vi "CR-导丝纤维毛发检测2.vi"(8 "error in (no error)":errorcluster caption="错误输入（无错误）", 11 "名称或相对路径":string="Template Program") -> (0 "error in (no error) 2":errorcluster caption="错误输入（无错误）")   [LabVIEW 2017]
uses:
  Global System.vi
  <vilib>/Utility/xml.llb/Write to XML File(string).vi
  Picture/SaveButtom.ctl
  <vilib>/vision/Pattern Matching.llb/IMAQ Curve Parameters.ctl
  <vilib>/userdefined/High Color/IMAQdx.ctl
panel:
  in  "相机选择":T1="cam0" caption="Session Out CCD3"
  in  "获取图像":bool
  in  "ROI获取":bool
  in  "创建模板":bool
  in  "保存图像":bool
  out "添加的路径":path
  in  "刷新":bool
  in  "测试按钮":bool
  in  "保存按钮":bool
  in  "Main":enum32{"主参数", "模板匹配参数 ", "测试效果"}(tab)
  in  "导丝纤维毛发检测2基础参数":T2={"IsNorImage"=TRUE, "Exposure Values"=100289, "ImagePath"=path "C:/Users/hedongpo/Desktop/514-hdp/Alignment Assemble System/Test Picture/B/3.bmp"} caption="参数界面" {"Exposure Values" scale=0.0..200000.0}
  in  "导丝纤维毛发检测2参数":T4={"Max Number"=11.0, "Curve Extraction Settings "={"Extraction Mode"=0, "Edge Threshold"=25, "Edge Filter Size"=1, "Min Length"=19, "Row Search Step Size"=5, "Col Search Step Size"=5, "Max Endpoint Gap"=10, "Closed"=FALSE, "Subpixel"=FALSE}, "Color Mode (Histogram 1)"=0, "Range (Threshold 1)"={"Lower value"=62.0, "Upper value"=255.0}, "Clamp Settings (Max Clamp 1)"={"Angle Range (+/-)"=10.0, "Edge Polarity"={"Start"=0, "End"=0}}} {"Clamp Settings (Max Clamp 1)"."Edge Polarity"."Start" items=["Any", "Rising", "Falling"]; "Clamp Settings (Max Clamp 1)"."Edge Polarity"."End" items=["Any", "Rising", "Falling"]; "Color Mode (Histogram 1)" items=["RGB", "HSL", "HSV", "HSI"]; "Curve Extraction Settings"."Extraction Mode" items=["Normal", "Uniform Regions"]; "Curve Extraction Settings"."Edge Filter Size" items=["Fine", "Normal", "Contour Tracing"]; "Curve Extraction Settings"."Max Endpoint Gap" min=0; "Curve Extraction Settings"."Col Search Step Size" min=1 max=255 step=1; "Curve Extraction Settings"."Row Search Step Size" min=1 max=255 step=1; "Curve Extraction Settings"."Min Length" min=0; "Curve Extraction Settings"."Edge Threshold" min=1 max=350 step=1}
  out "结果":bool
  out "原始图像":T5(plugin-control)
  out "路径输出":path
  in  "Vision Paramter Save Buttom":T6
  out "system time":string
  in  "取消按钮":bool
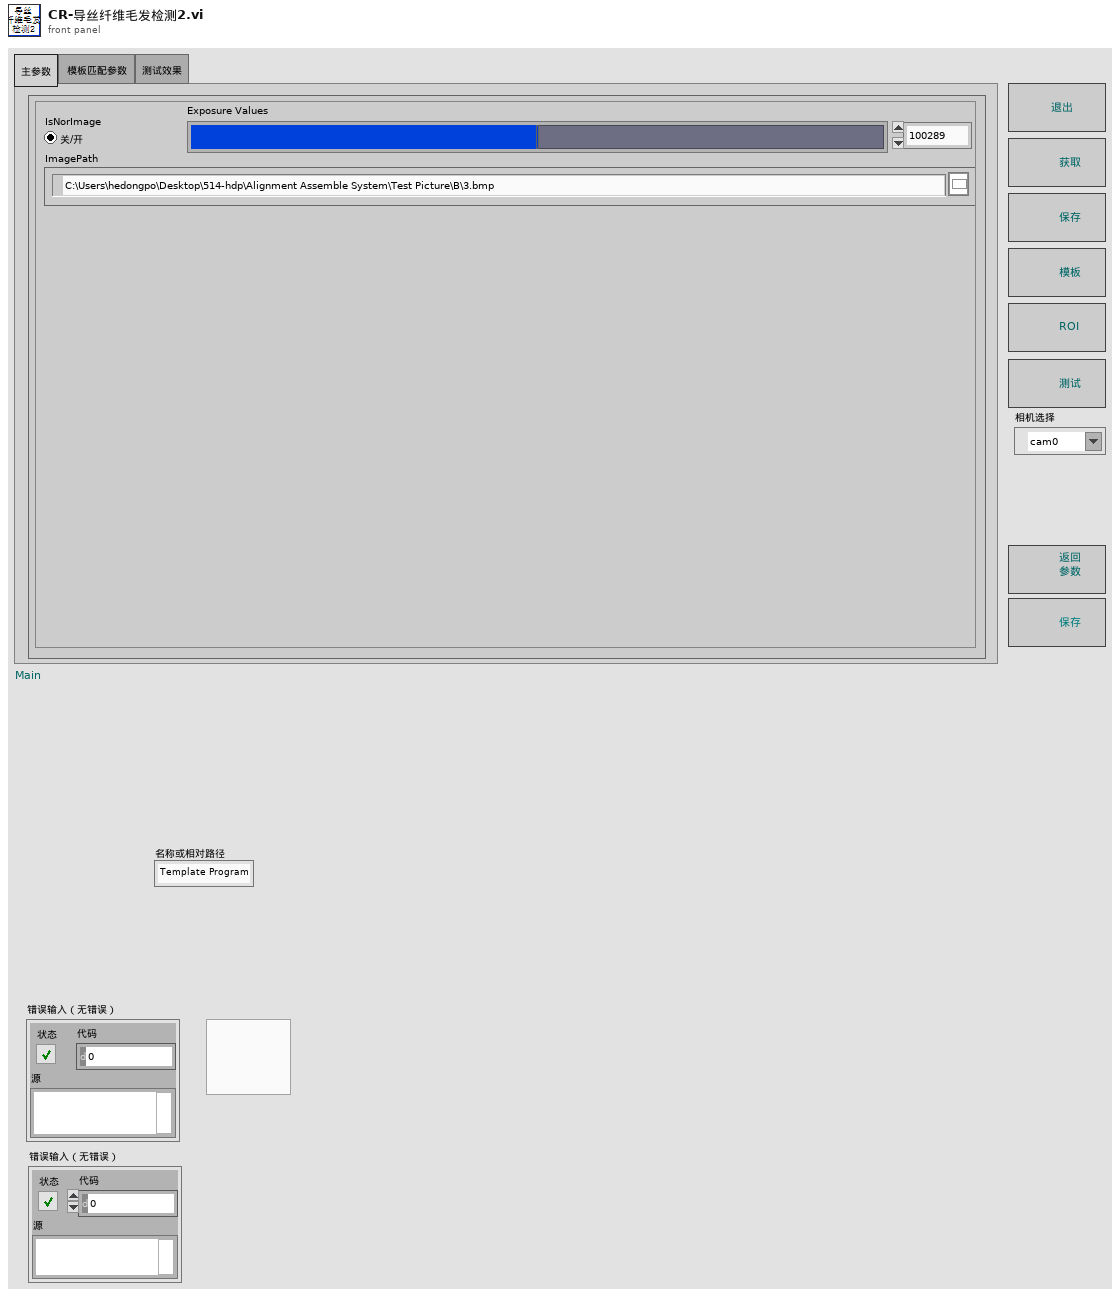
[diagram p1: front panel]
types:
  T1 = typedef "IMAQdx.ctl" = refnum<k21>
  T2 = cluster{"IsNorImage":bool, "Exposure Values":u32, "ImagePath":path}
  T3 = typedef "IMAQ Curve Parameters.ctl" = cluster{"Extraction Mode":u32, "Edge Threshold":i32, "Edge Filter Size":u32, "Min Length":i32, "Row Search Step Size":i32, "Col Search Step Size":i32, "Max Endpoint Gap":i32, "Closed":bool, "Subpixel":bool}
  T4 = cluster{"Max Number":sgl, "Curve Extraction Settings ":T3, "Color Mode (Histogram 1)":u16, "Range (Threshold 1)":cluster{"Lower value":sgl, "Upper value":sgl}, "Clamp Settings (Max Clamp 1)":cluster{"Angle Range (+/-)":dbl, "Edge Polarity":cluster{"Start":u32, "End":u32}}}
  T5 = typedef "IMAQ Image.ctl" = refnum<image>
  T6 = typedef "SaveButtom.ctl" = bool
  T7 = cluster{"index":i32, "this vi":refnum<vi>, "error out":errorcluster}
  T8 = cluster{"master data":string, "priority":u16, "secondary data":string[]}
  T9 = cluster{"case name":string[], "queue array":refnum<queue>[]}
  T10 = cluster{"Global Rectangle":i32[], "Contours":cluster{"Contour Type":u32, "ROI Type":u32, "Points":i32[]}[]}
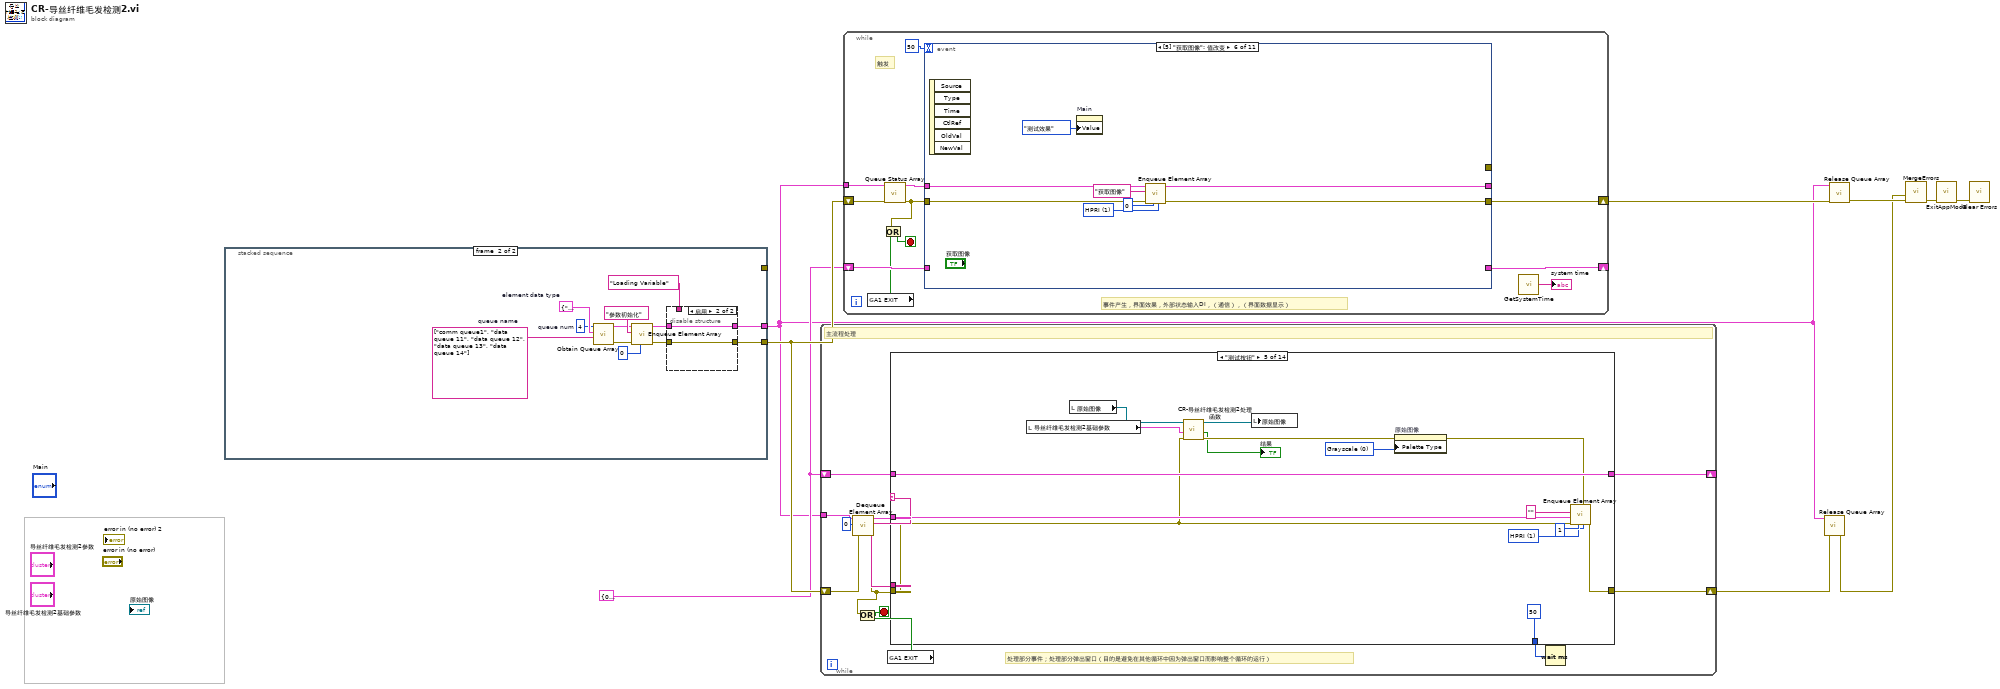
[diagram p0: block diagram]
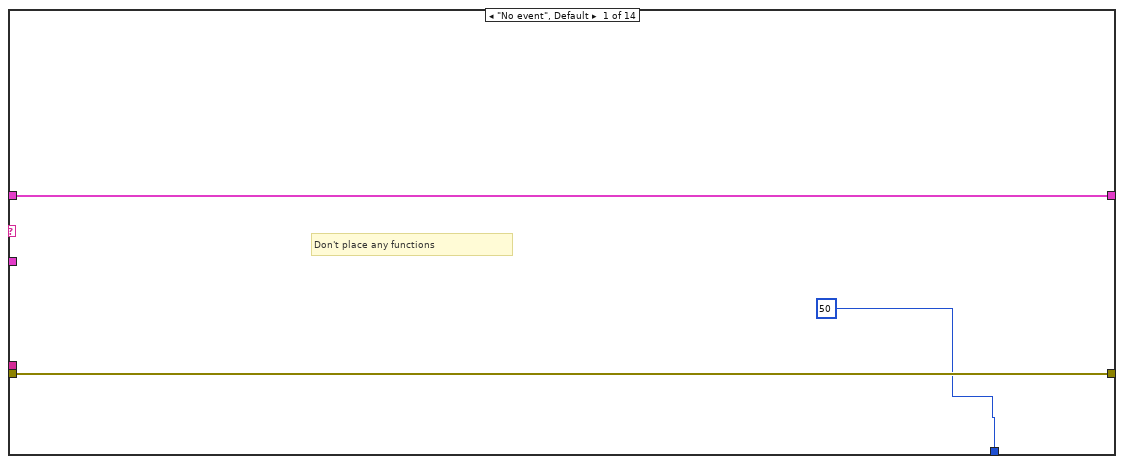
[diagram p2: hidden frame]
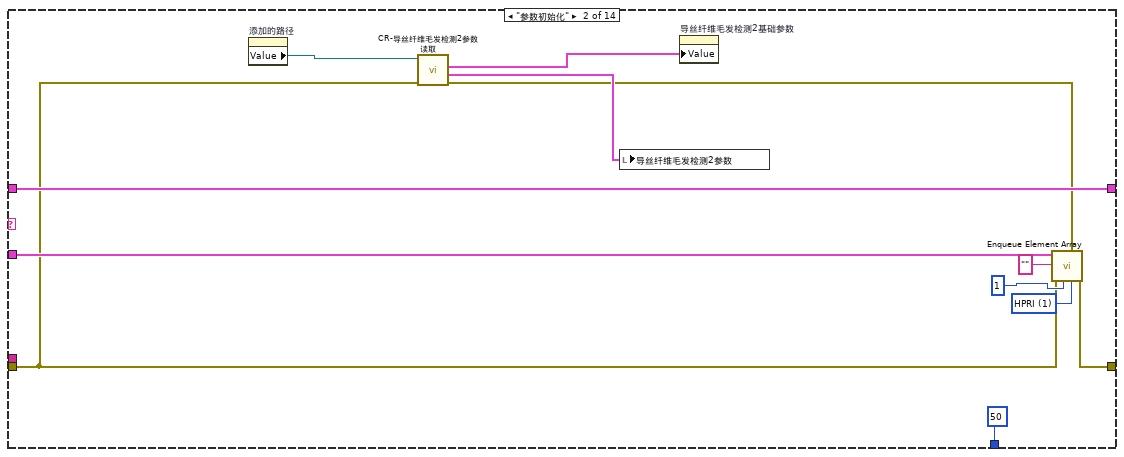
[diagram p3: hidden frame]
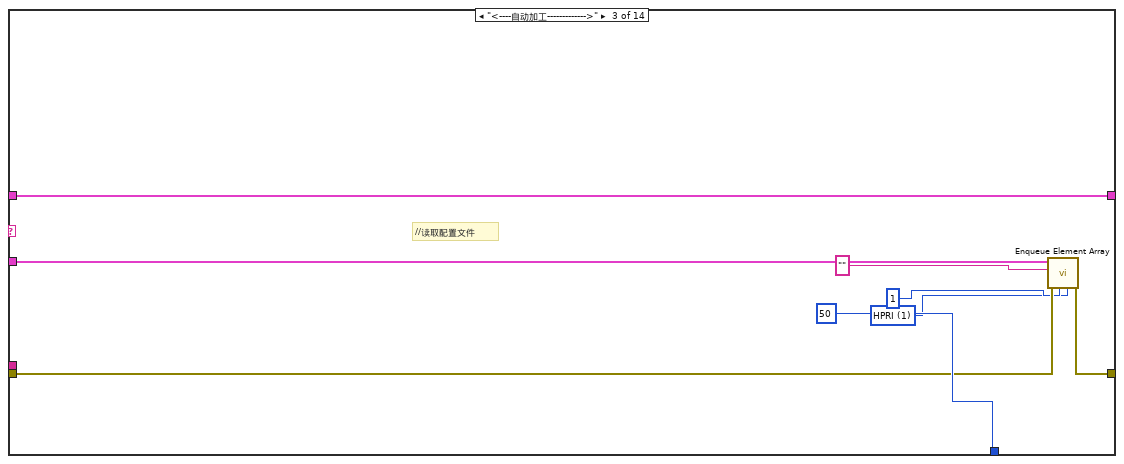
[diagram p4: hidden frame]
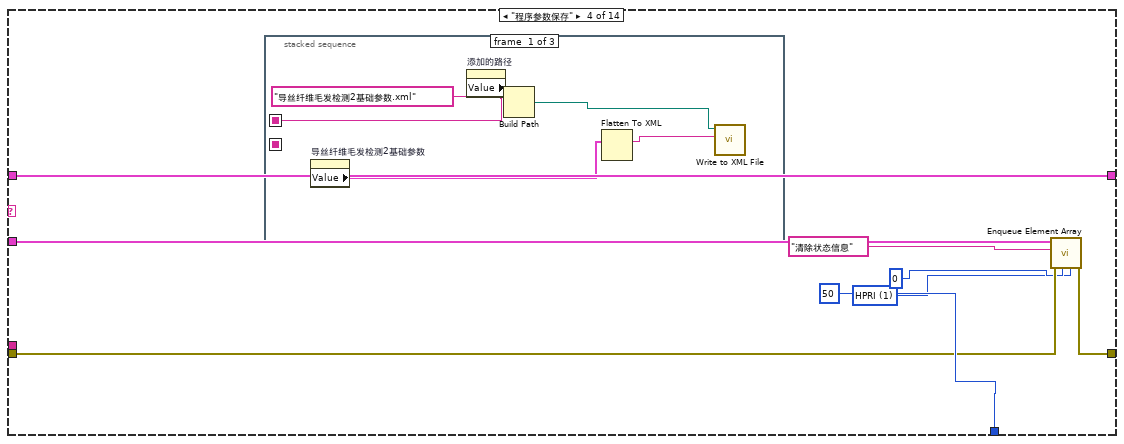
[diagram p5: hidden frame]
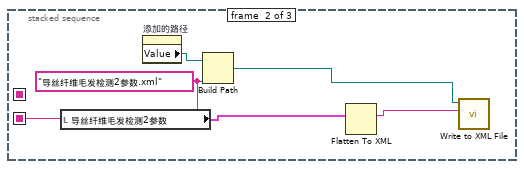
[diagram p6: hidden frame]
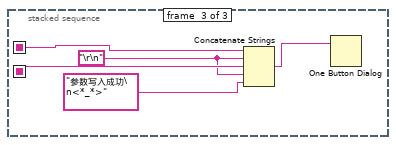
[diagram p7: hidden frame]
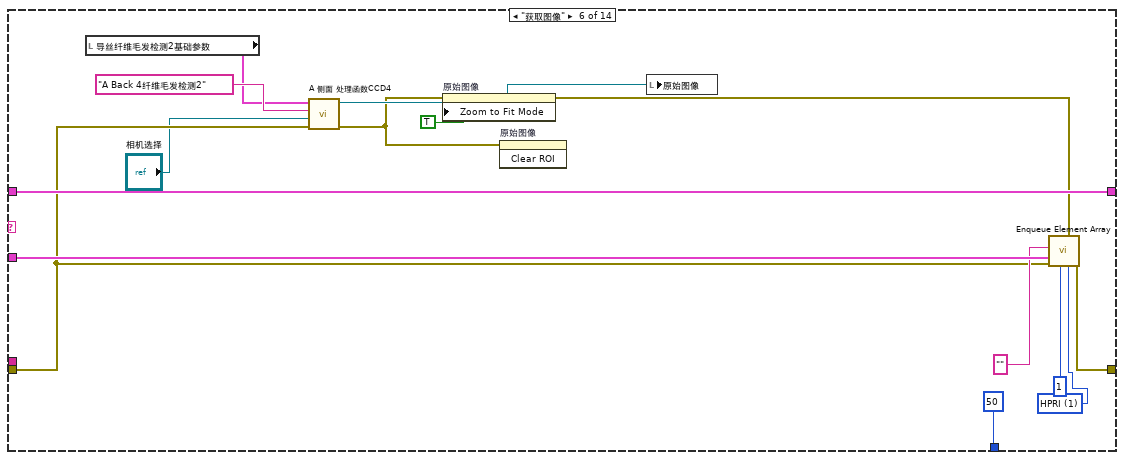
[diagram p8: hidden frame]
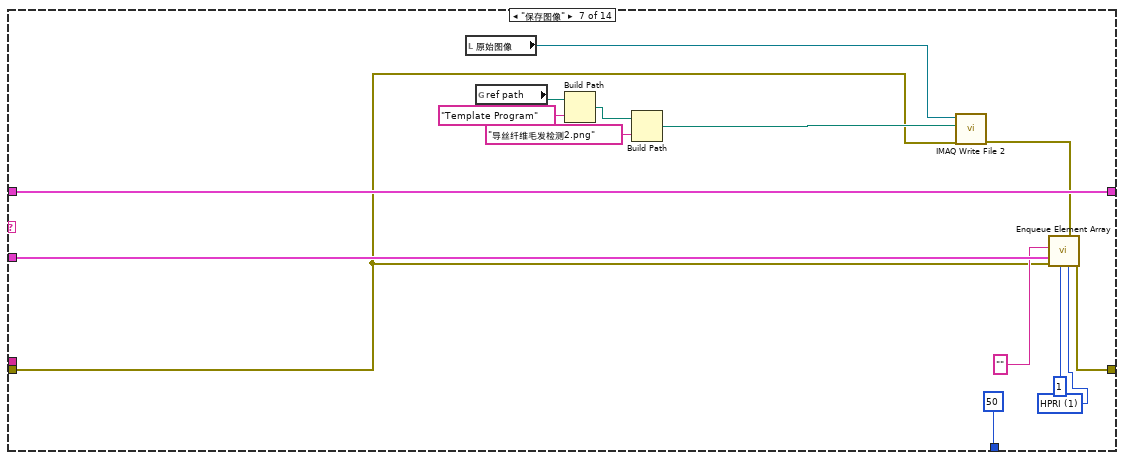
[diagram p9: hidden frame]
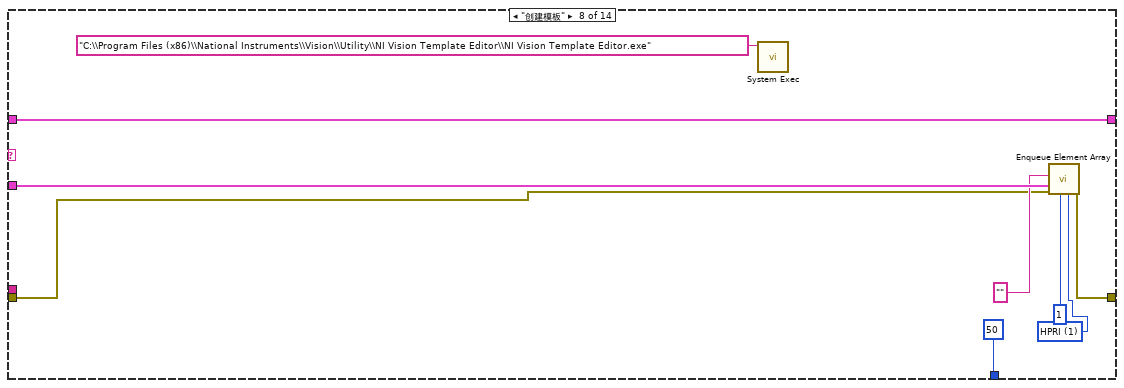
[diagram p10: hidden frame]
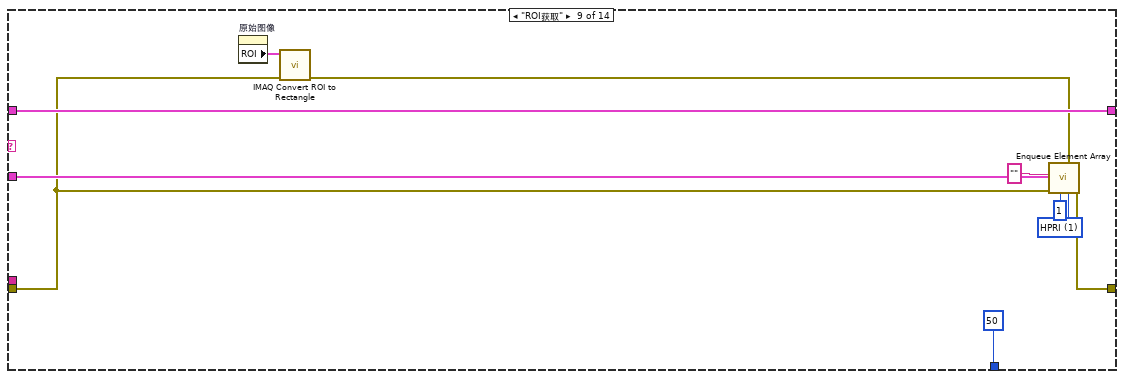
[diagram p11: hidden frame]
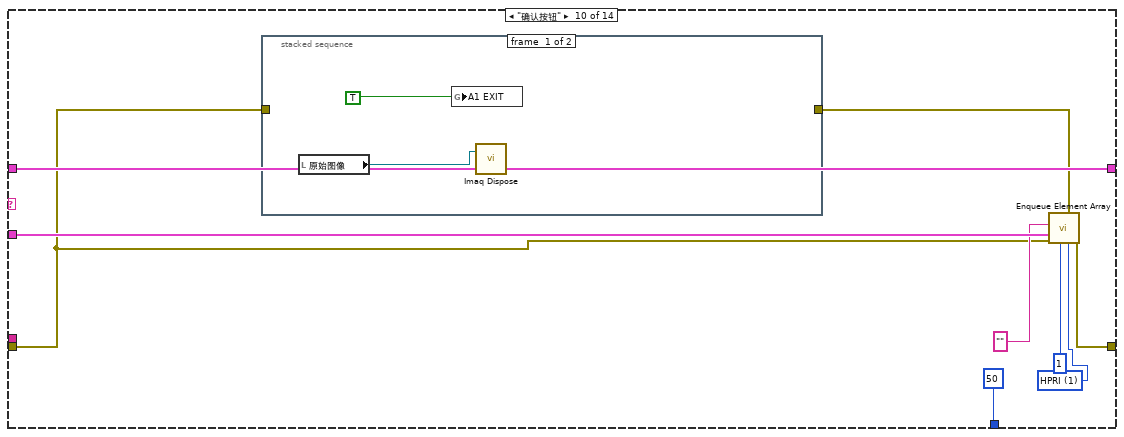
[diagram p12: hidden frame]
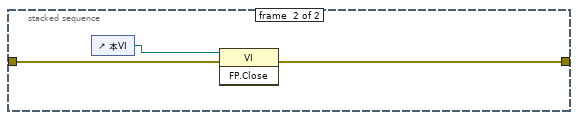
[diagram p13: hidden frame]
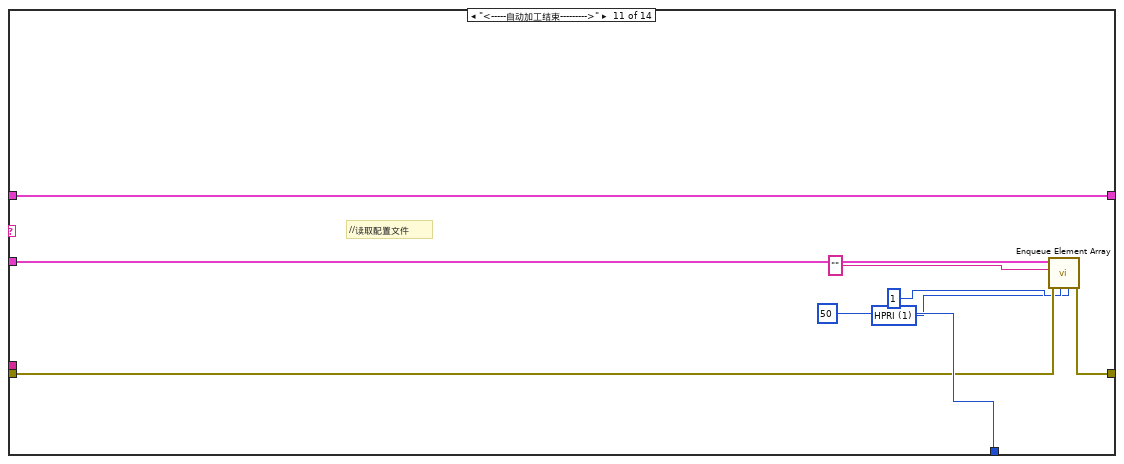
[diagram p14: hidden frame]
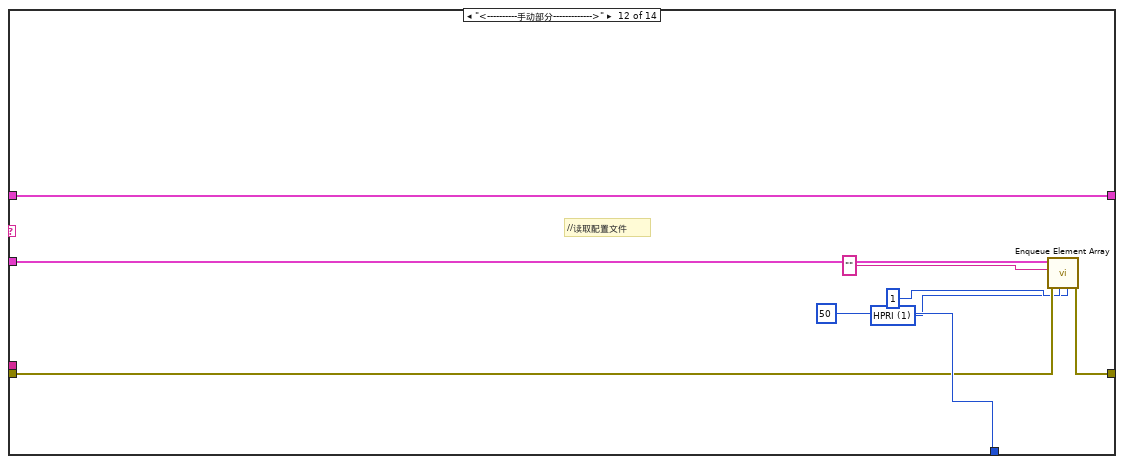
[diagram p15: hidden frame]
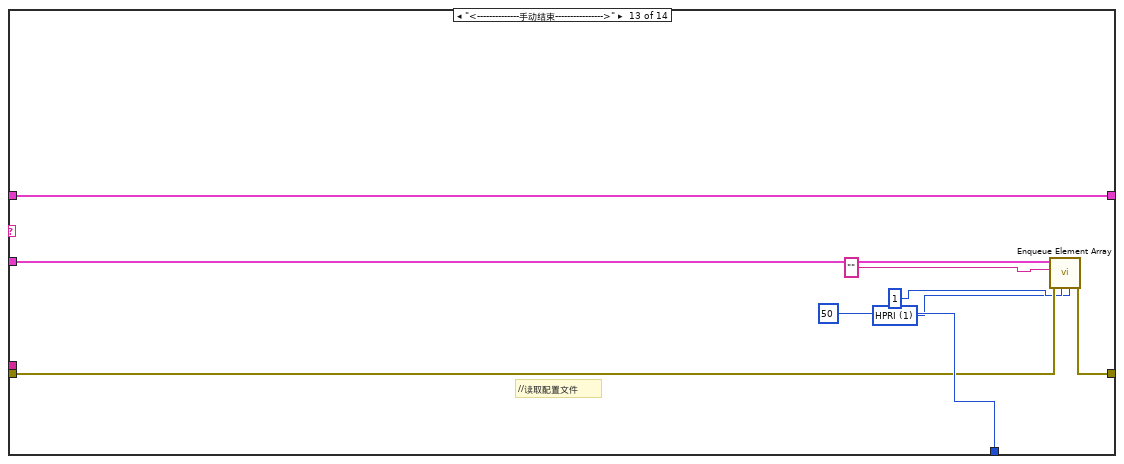
[diagram p16: hidden frame]
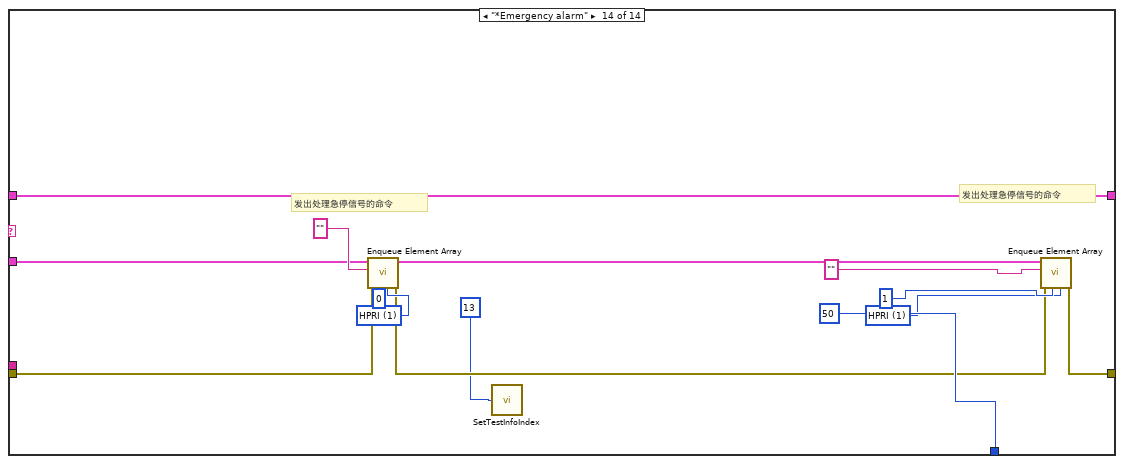
[diagram p17: hidden frame]
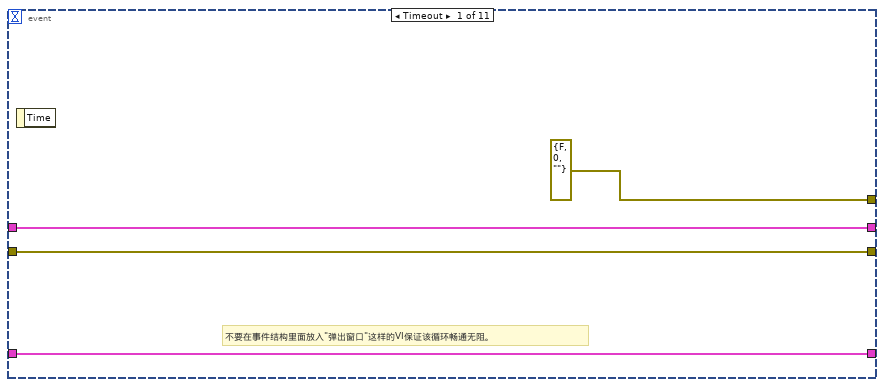
[diagram p18: hidden frame]
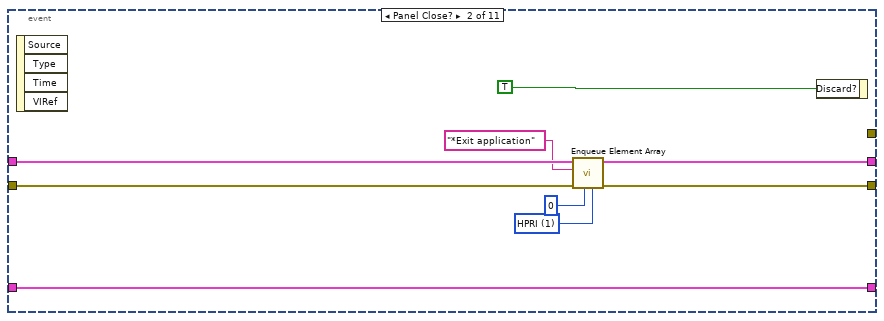
[diagram p19: hidden frame]
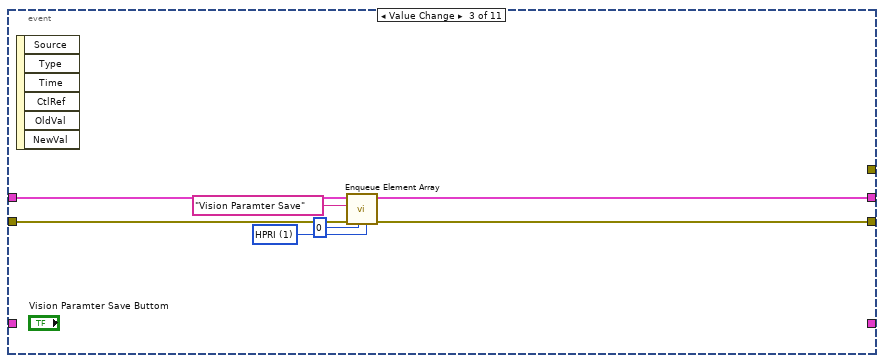
[diagram p20: hidden frame]
diagram:
  w4 = T7 {"index"=0, "this vi"=refnum, "error out"={"status"=FALSE, "code"=0, "source"=""}} ("parameter buffer")
  n1 = stacked-sequence {
    tunnel: [w15 _] -> _
    tunnel: [_ w19] -> w5
    tunnel: [_ w18] -> w1
    frame #0 {
      n2 = global read "Global System.vi" "ref path"() -> (w13:path)
      n3 = Build Path(base path=w13, name or relative path="Template Program" ("名称或相对路径")) -> (appended path=w11:path)
      n4 = property on="Main" class="TabCtl (严格)"("Value"=enum32{"主参数", "模板匹配参数 ", "测试效果"}."主参数" ("Main")) -> ()  [unwired: 2 in, 2 out]
      n5 = Build Path(base path=w11, name or relative path="名称或相对路径") -> (appended path=w17:path)
      "添加的路径" <- w17
      n6 = List Folder(path=w17) -> (path out=→"路径输出":path, error out=w15:errorcluster)  [unwired: 3 in, 2 out]
    }
    frame #1 {
      w27 = string[] ["comm queue1", "data queue 11", "data queue 12", "data queue 13", "data queue 14"]  # queue name
      w28 = 4  # queue num
      w29 = T8 {"master data"="", "priority"=0, "secondary data"=[]}  # element data type
      n7 = call "Obtain Queue Array.vi"("queue name"=w27, "element data type"=w29, "queue num"=w28) -> ("error out"=w23:errorcluster, "queue out"=w24:T9)  [unwired: 2 in, 1 out]
      n8 = call "Enqueue Element Array.vi"("queue index"=0, "error in"=w23, "master data"="参数初始化", "queue in"=w24) -> ("error out"=w22:errorcluster, "queue out"=w21:T9)  [unwired: 6 in]
      n9 = disable-structure shown="启用" {
        disable-tunnel: w22 -> [w35 w36]
        disable-tunnel: w21 -> [w34 w37]
        disable-tunnel: "Loading Variable" ("master data") -> [w33 _]
        disable-tunnel: [w31 w36] -> w19
        disable-tunnel: [w30 w37] -> w18
        frame Disabled {
          n10 = call "Enqueue Element Array.vi"("queue index"=12, "error in"=w35, "master data"=w33, "queue in"=w34) -> ("error out"=w31:errorcluster, "queue out"=w30:T9)  [unwired: 6 in]
        }
        frame Enabled {
        }
      }
    }
  }
  n11 = while {
    shift-right: [w50] -> w3
    shift-left: w5 -> [w41]
    shift-right: [w47] -> _
    shift-left: w4 -> [w48]
    tunnel: w1 -> [w43]
    stop <- w38 stop-if-true
    # "处理部分事件；处理部分弹出窗口（目的是避免在其他循环中因为弹出窗口而影响整个循环的运行）"
    # "主流程处理"
    n12 = call "Dequeue Element Array.vi"("queue in"=w43, "queue index"=0, "error in"=w41) -> ("queue out"=w46:T9, "master data"=w45:string, "secondary data"=w44:string[], "error out"=w40:errorcluster)  [unwired: 2 in, 1 out]
    n13 = global read "Global System.vi" "A1 EXIT"() -> (w39:bool)
    n14 = Or(x=w40, y=w39) -> (x .or. y?=w38:bool)
    n15 = case shown="\"测试按钮\"" w45 {
      tunnel: w46 -> [_ w64 w72 w74 w110 w125 w140 w149 w159 w168 w181 w189 w197 w203]
      tunnel: w40 -> [w52 w55 w68 w78 w104 w116 w127 w143 w152 w162 w177 w185 w193 w200]
      tunnel: [w52 w63 w71 w80 w109 w124 w139 w148 w158 w167 w180 w188 w196 w211] -> w50
      tunnel: [50 50 50 50 50 50 50 50 50 50 50 50 50 50] -> w49
      tunnel: w48 -> [w53 w60 w69 w75 w105 w120 w135 w144 w154 w163 w178 w186 w194 w209]
      tunnel: [w53 w60 w69 w75 w105 w120 w135 w144 w154 w163 w178 w186 w194 w209] -> w47
      tunnel: w44 -> [_ _ _ _ _ _ _ _ _ _ _ _ _ _]
      frame "No event", Default {
        # "Don't place any functions"
      }
      frame "参数初始化" {
        w59 = u16 1 items=["HPRI"=1, "LPRI"=0] ("priority")
        n16 = property on="添加的路径" class="Path"() -> ("Value"=w58:path)  [unwired: 2 in, 2 out]
        n17 = call "CR-导丝纤维毛发检测2参数读取.vi"("error in (no error)"=w55, "基路径"=w58) -> ("error out"=w54:errorcluster, "导丝纤维毛发检测2参数"=w56:T4, "导丝纤维毛发检测2基础参数"=w57:T2)  [unwired: 6 in]
        n18 = local write "导丝纤维毛发检测2参数"(w56) -> ()
        n19 = property on="导丝纤维毛发检测2基础参数" class="Clust (严格)"("Value"=w57) -> ()  [unwired: 2 in, 2 out]
        n20 = call "Enqueue Element Array.vi"("priority"=w59, "device error in"=w54, "queue index"=1, "error in"=w55, "master data"="" ("Element 1"), "queue in"=w64) -> ("error out"=w63:errorcluster)  [unwired: 4 in, 1 out]
      }
      frame "<----自动加工------------->" {
        w66 = u16 1 items=["HPRI"=1, "LPRI"=0] ("priority")
        # "//读取配置文件"
        n21 = call "Enqueue Element Array.vi"("priority"=w66, "queue index"=1, "error in"=w68, "master data"="" ("Element 1"), "queue in"=w72) -> ("error out"=w71:errorcluster)  [unwired: 5 in, 1 out]
      }
      frame "程序参数保存" {
        w76 = u16 1 items=["HPRI"=1, "LPRI"=0] ("priority")
        n22 = stacked-sequence {
          seq-local: [w82 _ _] -> [_ _ w95]
          seq-local: [_ w88 _] -> [_ _ w93]
          frame #0 {
            w82 = "导丝纤维毛发检测2基础参数.xml" ("名称或相对路径")
            n23 = property on="导丝纤维毛发检测2基础参数" class="Clust (严格)"() -> ("Value"=w85:T2)  [unwired: 2 in, 2 out]
            n24 = property on="添加的路径" class="Path"() -> ("Value"=w86:path)  [unwired: 2 in, 2 out]
            n25 = Build Path(base path=w86, name or relative path=w82) -> (appended path=w83:path)
            n26 = Flatten To XML(anything=w85) -> (xml string=w84:string)
            n27 = call-poly <vilib>:"Write to XML File.vi"("XML Input"=w84, "XML File Path"=w83) -> ()  [unwired: 7 in, 3 out]
          }
          frame #1 {
            w88 = "导丝纤维毛发检测2参数.xml" ("名称或相对路径")
            n28 = local read "导丝纤维毛发检测2参数"() -> (w87:T4)
            n29 = property on="添加的路径" class="Path"() -> ("Value"=w91:path)  [unwired: 2 in, 2 out]
            n30 = Build Path(base path=w91, name or relative path=w88) -> (appended path=w89:path)
            n31 = Flatten To XML(anything=w87) -> (xml string=w90:string)
            n32 = call-poly <vilib>:"Write to XML File.vi"("XML Input"=w90, "XML File Path"=w89) -> ()  [unwired: 7 in, 3 out]
          }
          frame #2 {
            w92 = "\r\n"
            n33 = Concatenate Strings(w95, w92, w93, w92, "参数写入成功\n<*_*>" ("消息")) -> (w94:string)
            n34 = One Button Dialog(message=w94) -> ()  [unwired: 1 in, 1 out]
          }
        }
        n35 = call "Enqueue Element Array.vi"("priority"=w76, "queue index"=0, "error in"=w78, "master data"="清除状态信息" ("Element 1"), "queue in"=w74) -> ("error out"=w80:errorcluster)  [unwired: 5 in, 1 out]
      }
      frame "测试按钮" {
        w100 = u32 0 items=["Grayscale", "Binary", "Gradient", "Rainbow", "Temperature", "User Defined", "Binary 16 Bit", "Gradient 16 Bit", "Rainbow 16 Bit", "Temperature 16 Bit", "User Defined 16 Bit"] ("Palette:Palette Type")
        w106 = u16 1 items=["HPRI"=1, "LPRI"=0] ("priority")
        n36 = local read "导丝纤维毛发检测2基础参数"() -> (w97:T2)
        n37 = local read "原始图像"() -> (w102:T5)
        n38 = call "CR-导丝纤维毛发检测2处理函数.vi"("error in (no error)"=w104, "导丝纤维毛发检测2基础参数"=w97, "Image in"=w102) -> ("error out"=w101:errorcluster, "纤维毛发"=→"结果":bool, "Image out"=w103:T5)  [unwired: 5 in, 1 out]
        n39 = local write "原始图像"(w103) -> ()
        n40 = property on="原始图像" class="ImageControl"(error in=w101, "Palette Type"=w100) -> (error out=w99:errorcluster)  [unwired: 1 in, 1 out]
        n41 = call "Enqueue Element Array.vi"("priority"=w106, "device error in"=w99, "queue index"=1, "error in"=w104, "master data"="" ("Element 1"), "queue in"=w110) -> ("error out"=w109:errorcluster)  [unwired: 4 in, 1 out]
      }
      frame "获取图像" {
        w121 = u16 1 items=["HPRI"=1, "LPRI"=0] ("priority")
        n42 = local read "导丝纤维毛发检测2基础参数"() -> (w118:T2)
        n43 = call "A 侧面 处理函数CCD4.vi"("error in (no error)"=w116, "相机选择"="相机选择", "New Image"="A Back 4纤维毛发检测2" ("Image Name"), "ParamsUI"=w118) -> ("error out"=w113:errorcluster, "Image out"=w117:T5)  [unwired: 4 in, 2 out]
        n44 = property on="原始图像" class="ImageControl"(error in=w113, "Zoom to Fit Mode"=TRUE) -> (error out=w114:errorcluster)  [unwired: 1 in, 1 out]
        n45 = invoke on="原始图像" class="ImageControl" method="Clear ROI"(error in=w113) -> ()  [unwired: 2 in, 3 out]
        n46 = local write "原始图像"(w117) -> ()
        n47 = call "Enqueue Element Array.vi"("priority"=w121, "device error in"=w114, "queue index"=1, "error in"=w116, "master data"="" ("Element 1"), "queue in"=w125) -> ("error out"=w124:errorcluster)  [unwired: 4 in, 1 out]
      }
      frame "保存图像" {
        w136 = u16 1 items=["HPRI"=1, "LPRI"=0] ("priority")
        n48 = local read "原始图像"() -> (w128:T5)
        n49 = global read "Global System.vi" "ref path"() -> (w134:path)
        n50 = Build Path(base path=w134, name or relative path="Template Program" ("名称或相对路径")) -> (appended path=w132:path)
        n51 = Build Path(base path=w132, name or relative path="导丝纤维毛发检测2.png" ("名称或相对路径")) -> (appended path=w130:path)
        n52 = call-poly "IMAQ Write File 2"("error in (no error)"=w127, "File Path"=w130, "Image"=w128) -> ("error out"=w129:errorcluster)  [unwired: 7 in, 1 out]
        n53 = call "Enqueue Element Array.vi"("priority"=w136, "device error in"=w129, "queue index"=1, "error in"=w127, "master data"="" ("Element 1"), "queue in"=w140) -> ("error out"=w139:errorcluster)  [unwired: 4 in, 1 out]
      }
      frame "创建模板" {
        w145 = u16 1 items=["HPRI"=1, "LPRI"=0] ("priority")
        n54 = call <vilib>:"System Exec.vi"("command line"="C:\\Program Files (x86)\\National Instruments\\Vision\\Utility\\NI Vision Template Editor\\NI Vision Template Editor.exe") -> ()  [unwired: 7 in, 4 out]
        n55 = call "Enqueue Element Array.vi"("priority"=w145, "queue index"=1, "error in"=w143, "master data"="" ("Element 1"), "queue in"=w149) -> ("error out"=w148:errorcluster)  [unwired: 5 in, 1 out]
      }
      frame "ROI获取" {
        w155 = u16 1 items=["HPRI"=1, "LPRI"=0] ("priority")
        n56 = property on="原始图像" class="ImageControl"() -> ("ROI"=w153:T10)  [unwired: 2 in, 2 out]
        n57 = call "IMAQ Convert ROI to Rectangle"("error in (no error)"=w152, "ROI Descriptor"=w153) -> ("error out"=w151:errorcluster)  [unwired: 7 in, 1 out]
        n58 = call "Enqueue Element Array.vi"("priority"=w155, "device error in"=w151, "queue index"=1, "error in"=w152, "master data"="" ("Element 1"), "queue in"=w159) -> ("error out"=w158:errorcluster)  [unwired: 4 in, 1 out]
      }
      frame "确认按钮" {
        w164 = u16 1 items=["HPRI"=1, "LPRI"=0] ("priority")
        n59 = stacked-sequence {
          tunnel: w162 -> [_ w173]
          tunnel: [_ w172] -> w161
          frame #0 {
            n60 = local read "原始图像"() -> (w170:T5)
            n61 = global write "Global System.vi" "A1 EXIT"(TRUE ("EXIT")) -> ()
            n62 = call "Imaq Dispose"("Image"=w170) -> ()  [unwired: 5 in, 1 out]
          }
          frame #1 {
            n63 = control-ref of="本VI"() -> (w174:refnum<vi>)
            n64 = invoke class="VI" method="FP.Close"(reference=w174, error in=w173) -> (error out=w172:errorcluster)  [unwired: 1 in, 2 out]
          }
        }
        n65 = call "Enqueue Element Array.vi"("priority"=w164, "device error in"=w161, "queue index"=1, "error in"=w162, "master data"="" ("Element 1"), "queue in"=w168) -> ("error out"=w167:errorcluster)  [unwired: 4 in, 1 out]
      }
      frame "<-----自动加工结束--------->" {
        w175 = u16 1 items=["HPRI"=1, "LPRI"=0] ("priority")
        # "//读取配置文件"
        n66 = call "Enqueue Element Array.vi"("priority"=w175, "queue index"=1, "error in"=w177, "master data"="" ("Element 1"), "queue in"=w181) -> ("error out"=w180:errorcluster)  [unwired: 5 in, 1 out]
      }
      frame "<----------手动部分------------->" {
        w183 = u16 1 items=["HPRI"=1, "LPRI"=0] ("priority")
        # "//读取配置文件"
        n67 = call "Enqueue Element Array.vi"("priority"=w183, "queue index"=1, "error in"=w185, "master data"="" ("Element 1"), "queue in"=w189) -> ("error out"=w188:errorcluster)  [unwired: 5 in, 1 out]
      }
      frame "<--------------手动结束---------------->" {
        w191 = u16 1 items=["HPRI"=1, "LPRI"=0] ("priority")
        # "//读取配置文件"
        n68 = call "Enqueue Element Array.vi"("priority"=w191, "queue index"=1, "error in"=w193, "master data"="" ("Element 1"), "queue in"=w197) -> ("error out"=w196:errorcluster)  [unwired: 5 in, 1 out]
      }
      frame "*Emergency alarm" {
        w206 = u16 1 items=["HPRI"=1, "LPRI"=0] ("priority")
        w207 = u16 1 items=["HPRI"=1, "LPRI"=0] ("priority")
        # "发出处理急停信号的命令"
        # "发出处理急停信号的命令"
        n69 = call "Enqueue Element Array.vi"("priority"=w206, "queue index"=0, "error in"=w200, "master data"="" ("Element 1"), "queue in"=w203) -> ("error out"=w201:errorcluster, "queue out"=w202:T9)  [unwired: 5 in]
        n70 = call "SetTestInfoIndex.vi"("test info index"=13) -> ()
        n71 = call "Enqueue Element Array.vi"("priority"=w207, "queue index"=1, "error in"=w201, "master data"="" ("Element 1"), "queue in"=w202) -> ("error out"=w211:errorcluster)  [unwired: 5 in, 1 out]
      }
    }
    n72 = Wait (ms)(milliseconds to wait=w49) -> ()  [unwired: 1 out]
  }
  n73 = while {
    shift-right: [w216] -> w6
    shift-left: w5 -> [w220]
    shift-right: [w218] -> _
    shift-left: w4 -> [w219]
    tunnel: w1 -> [w222]
    stop <- w213 stop-if-true
    # "触发"
    # "事件产生，界面效果，外部状态输入DI，（通信），（界面数据显示）"
    n74 = global read "Global System.vi" "A1 EXIT"() -> (w214:bool)
    n75 = call "Queue Status Array.vi"("error in (no error)"=w220, "queue in"=w222) -> ("error out"=w215:errorcluster, "queue out"=w217:T9)  [unwired: 4 in]
    n76 = Or(x=w215, y=w214) -> (x .or. y?=w213:bool)
    n77 = event shown="[5] \"获取图像\": 值改变" {
      selector: _ -> [_ _ _ _ _ _ _ _ _ _ _]
      dyn-events: _ -> [_ _ _ _ _ _ _ _ _ _ _]
      timeout: 50 -> [_ _ _ _ _ _ _ _ _ _ _]
      tunnel: w219 -> [w227 w235 _ _ _ _ _ _ _ _ _]
      tunnel: [w227 w235 _ _ _ _ _ _ _ _ _] -> w218
      tunnel: [errorcluster {"status"=FALSE, "code"=0, "source"=""} ("error out") _ _ _ _ _ _ _ _ _ _] -> _
      tunnel: w217 -> [w225 w234 w240 w247 w254 w262 w269 w276 w284 w292 w300]
      tunnel: w215 -> [w224 w233 w239 w246 w253 w261 w268 w275 w283 w291 w299]
      tunnel: [w224 w232 w237 w244 w251 w259 w266 w273 w281 w289 w297] -> w216
      tunnel: [w225 w231 w238 w245 w252 w260 w267 w274 w282 w290 w298] -> _
      event Timeout {
        # "不要在事件结构里面放入\"弹出窗口\"这样的VI保证该循环畅通无阻。"
        n78 = event-data() -> ()  [unwired: 1 in, 1 out]
      }
      event Panel Close? {
        w229 = u16 1 items=["HPRI"=1, "LPRI"=0] ("priority")
        n79 = event-data() -> ()  [unwired: 1 in, 4 out]
        n80 = call "Enqueue Element Array.vi"("priority"=w229, "queue index"=0, "error in"=w233, "master data"="*Exit application", "queue in"=w234) -> ("error out"=w232:errorcluster, "queue out"=w231:T9)  [unwired: 5 in]
        n81 = event-data("Discard?"=TRUE) -> ()  [unwired: 1 in, 1 out]
      }
      event Value Change {
        w242 = u16 1 items=["HPRI"=1, "LPRI"=0] ("priority")
        n82 = event-data() -> ()  [unwired: 1 in, 6 out]
        n83 = call "Enqueue Element Array.vi"("priority"=w242, "queue index"=0, "error in"=w239, "master data"="Vision Paramter Save", "queue in"=w240) -> ("error out"=w237:errorcluster, "queue out"=w238:T9)  [unwired: 5 in]
      }
      event "取消按钮": Value Change {
        w249 = u16 1 items=["HPRI"=1, "LPRI"=0] ("priority")
        n84 = event-data() -> ()  [unwired: 1 in, 6 out]
        n85 = call "Enqueue Element Array.vi"("priority"=w249, "queue index"=0, "error in"=w246, "master data"="确认按钮", "queue in"=w247) -> ("error out"=w244:errorcluster, "queue out"=w245:T9)  [unwired: 5 in]
      }
      event "保存按钮": Value Change {
        w256 = u16 1 items=["HPRI"=1, "LPRI"=0] ("priority")
        n86 = event-data() -> ()  [unwired: 1 in, 6 out]
        n87 = call "Enqueue Element Array.vi"("priority"=w256, "queue index"=0, "error in"=w253, "master data"="程序参数保存", "queue in"=w254) -> ("error out"=w251:errorcluster, "queue out"=w252:T9)  [unwired: 5 in]
      }
      event "获取图像": Value Change {
        w264 = u16 1 items=["HPRI"=1, "LPRI"=0] ("priority")
        n88 = event-data() -> ()  [unwired: 1 in, 6 out]
        n89 = property on="Main" class="TabCtl (严格)"("Value"=enum32{"主参数", "模板匹配参数 ", "测试效果"}."测试效果" ("Main")) -> ()  [unwired: 2 in, 2 out]
        n90 = call "Enqueue Element Array.vi"("priority"=w264, "queue index"=0, "error in"=w261, "master data"="获取图像", "queue in"=w262) -> ("error out"=w259:errorcluster, "queue out"=w260:T9)  [unwired: 5 in]
      }
      event "保存图像": Value Change {
        w271 = u16 1 items=["HPRI"=1, "LPRI"=0] ("priority")
        n91 = event-data() -> ()  [unwired: 1 in, 6 out]
        n92 = call "Enqueue Element Array.vi"("priority"=w271, "queue index"=0, "error in"=w268, "master data"="保存图像", "queue in"=w269) -> ("error out"=w266:errorcluster, "queue out"=w267:T9)  [unwired: 5 in]
      }
      event "创建模板": Value Change {
        w278 = u16 1 items=["HPRI"=1, "LPRI"=0] ("priority")
        n93 = event-data() -> ()  [unwired: 1 in, 6 out]
        n94 = call "Enqueue Element Array.vi"("priority"=w278, "queue index"=0, "error in"=w275, "master data"="创建模板", "queue in"=w276) -> ("error out"=w273:errorcluster, "queue out"=w274:T9)  [unwired: 5 in]
      }
      event "ROI获取": Value Change {
        w286 = u16 1 items=["HPRI"=1, "LPRI"=0] ("priority")
        n95 = event-data() -> ()  [unwired: 1 in, 6 out]
        n96 = property on="Main" class="TabCtl (严格)"("Value"=enum32{"主参数", "模板匹配参数 ", "测试效果"}."模板匹配参数 " ("Main")) -> ()  [unwired: 2 in, 2 out]
        n97 = call "Enqueue Element Array.vi"("priority"=w286, "queue index"=0, "error in"=w283, "master data"="ROI获取", "queue in"=w284) -> ("error out"=w281:errorcluster, "queue out"=w282:T9)  [unwired: 5 in]
      }
      event "测试按钮": Value Change {
        w294 = u16 1 items=["HPRI"=1, "LPRI"=0] ("priority")
        n98 = event-data() -> ()  [unwired: 1 in, 6 out]
        n99 = property on="Main" class="TabCtl (严格)"("Value"=enum32{"主参数", "模板匹配参数 ", "测试效果"}."测试效果" ("Main")) -> ()  [unwired: 2 in, 2 out]
        n100 = call "Enqueue Element Array.vi"("priority"=w294, "queue index"=0, "error in"=w291, "master data"="测试按钮", "queue in"=w292) -> ("error out"=w289:errorcluster, "queue out"=w290:T9)  [unwired: 5 in]
      }
      event "刷新": Value Change {
        n101 = event-data() -> ()  [unwired: 1 in, 6 out]
        n102 = disable-structure shown="禁用" {
          disable-tunnel: w300 -> [w304 _]
          disable-tunnel: w299 -> [w303 _]
          disable-tunnel: [w302 _] -> w298
          disable-tunnel: [w301 _] -> w297
          frame Disabled {
            w306 = u16 1 items=["HPRI"=1, "LPRI"=0] ("priority")
            # "刷新"
            n103 = call "Enqueue Element Array.vi"("priority"=w306, "queue index"=0, "error in"=w303, "master data"="刷新", "queue in"=w304) -> ("error out"=w301:errorcluster, "queue out"=w302:T9)  [unwired: 5 in]
          }
          frame Enabled {
          }
        }
        n104 = property on="Main" class="TabCtl (严格)"("Value"=enum32{"主参数", "模板匹配参数 ", "测试效果"}."模板匹配参数 " ("Main")) -> ()  [unwired: 2 in, 2 out]
      }
    }
    n105 = call "GetSystemTime.vi"() -> ("date/time string"=→"system time":string)  [unwired: 7 in]
  }
  n106 = call "Release Queue Array.vi"("error in"=w3, "queue in"=w1) -> ("error out"=w2:errorcluster)  [unwired: 2 in, 3 out]
  n107 = call "Release Queue Array.vi"("error in"=w6, "queue in"=w1) -> ("error out"=w9:errorcluster)  [unwired: 2 in, 3 out]
  n108 = call "MergeErrors.vi"("error in 3 (no error)"=w2, "error in 4 (no error)"=w9) -> ("error out"=w8:errorcluster)  [unwired: 6 in]
  n109 = call "ExitAppMode.vi"("error in (no error)"=w8) -> ("error out"=w7:errorcluster)  [unwired: 10 in]
  n110 = call <vilib>:"Clear Errors.vi"("error in (no error)"=w7) -> ()  [unwired: 5 in, 2 out]
